vi "Create Access Database.vi"(8 "错误输入（无错误）":errorcluster, 10 "Password":string, 11 "路径":path) -> (0 "错误输出":errorcluster, 3 "路径 out":path)   [LabVIEW 2016, in "Access Lib.lvlib"]
uses:
  Access Lib.lvlib
panel:
  # "使用ActiveX命令来创建新的Access数据库文件。\n     1.从ActiveX面板选择Automation Open VI打开一个\"Microsoft ADO Ext. x.x for DDL and Security Version x.x\"引用，其中x.x 代表版本号。 \n     2.右键单击选择Catalog对象。 \n     3.在程序框图放置一个方法节点并将之连接至Automation Open函数。右键单击 Method?Select Method选择Create方法。 \n     4.右键点击参数 Connect String输入选择 Create?Constant。输入字符串常量：Provider=Microsoft.Jet.OLEDB.4.0;Data Source=yourfilename.mdb;Mode=Share Deny Read|Share Deny Write;User ID=Admin;Jet OLEDB:Database Password=123456。 文件名是创建的Access数据库文件路径名\n指定文件路径：C:\\My Documents\\MyAccessDB.mdb\n指定以独占方式创建：Mode=Share Deny Read|Share Deny Write\n创建密码：User ID=Admin;Jet OLEDB:Database Password=123456；若Password为空则无密码"
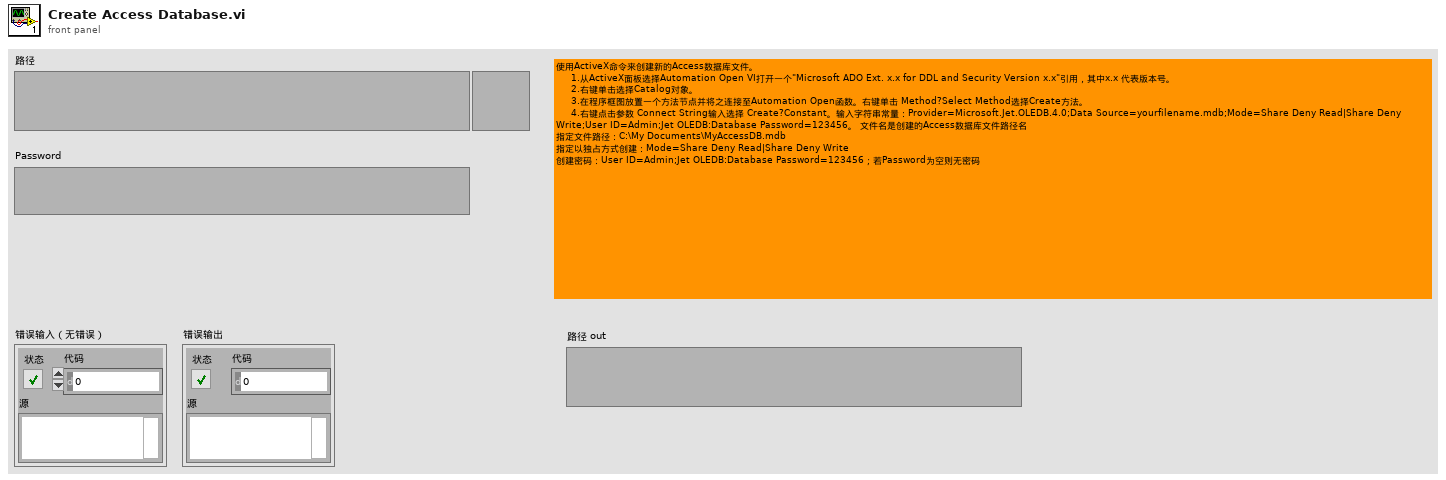
[diagram p1: front panel]
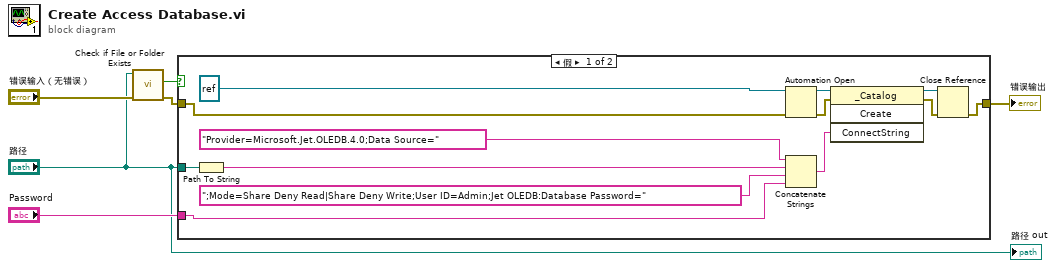
[diagram p0: block diagram]
diagram:
  n1 = call <vilib>:"Check if File or Folder Exists.vi"("error in (no error)"="错误输入（无错误）", "path"="路径") -> ("error out"=w3:errorcluster, "file or folder exists?"=w5:bool)  [unwired: 7 in, 1 out]
  n2 = case shown="假" w5 {
    tunnel: "Password" -> [w10 _]
    tunnel: "路径" -> [w11 _]
    tunnel: w3 -> [w8 w20]
    tunnel: [w7 w20] -> w2
    frame False {
      n3 = Path To String(path=w11) -> (string=w14:string)
      n4 = Automation Open(error in (no error)=w8, Automation Refnum=refnum<k7> refnum ("ADOX._Catalog")) -> (Automation Refnum=w19:refnum<k7>, error out=w17:errorcluster)  [unwired: 2 in]
      n5 = Concatenate Strings("Provider=Microsoft.Jet.OLEDB.4.0;Data Source=" ("ConnectString"), w14, ";Mode=Share Deny Read|Share Deny Write;User ID=Admin;Jet OLEDB:Database Password=" ("字符串"), w10) -> (w15:string)
      n6 = invoke on="调用节点" class="_Catalog" method="Create"(reference=w19, error in=w17, "ConnectString"=w15) -> (reference out=w18:refnum<k7>, error out=w16:errorcluster)  [unwired: 1 in, 2 out]
      n7 = Close Reference(reference=w18, error in (no error)=w16) -> (error out=w7:errorcluster)
    }
    frame True {
    }
  }
  "错误输出" <- w2
  "路径 out" <- "路径"
